vi "Update Array Ref.vi"(10 "%":dbl[](array[numeric]), 11 "appended array":refnum<vi>[](array[refnum])) -> ()   [LabVIEW 2018]
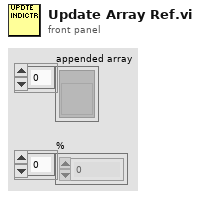
[diagram p1: front panel]
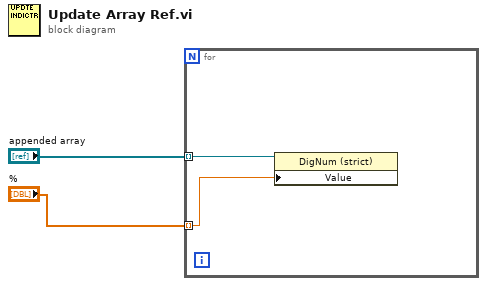
[diagram p0: block diagram]
diagram:
  n1 = for {
    tunnel: "appended array" -> [w4] mode=indexing
    tunnel: "%" -> [w3] mode=indexing
    n2 = property class="DigNum (strict)"(reference=w4, "Value"=w3) -> ()  [unwired: 1 in, 2 out]
  }
